vi "Sensors Modifications.vi"(1 "Sensors Global Values In":T1) -> (0 "Sensors Global Values Out":T1)   [LabVIEW 2013]
panel:
  in  "Sonar V/cm":dbl
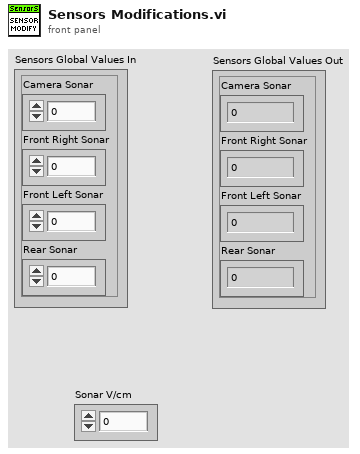
[diagram p1: front panel]
types:
  T1 = cluster{"Camera Sonar":dbl, "Front Right Sonar":dbl, "Front Left Sonar":dbl, "Rear Sonar":dbl}
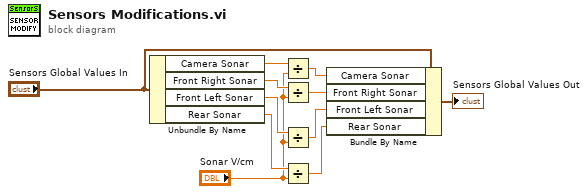
[diagram p0: block diagram]
diagram:
  n1 = Unbundle By Name("Sensors Global Values In") -> ("Camera Sonar"=w9:dbl, "Front Right Sonar"=w7:dbl, "Front Left Sonar"=w6:dbl, "Rear Sonar"=w5:dbl)
  n2 = Divide(x=w9, y="Sonar V/cm") -> (x/y=w8:dbl)
  n3 = Divide(x=w7, y="Sonar V/cm") -> (x/y=w3:dbl)
  n4 = Divide(x=w6, y="Sonar V/cm") -> (x/y=w2:dbl)
  n5 = Divide(x=w5, y="Sonar V/cm") -> (x/y=w1:dbl)
  n6 = Bundle By Name(cluster="Sensors Global Values In", "Camera Sonar"=w8, "Front Right Sonar"=w3, "Front Left Sonar"=w2, "Rear Sonar"=w1) -> (→"Sensors Global Values Out":T1)
